vi "practica15RNAtarea.vi"() -> ()   [LabVIEW 2017]
uses:
  <vilib>/Analysis/Matrix/Datatypes/RealMatrix.ctl
  <vilib>/Analysis/Matrix/Numeric/Multiply/Multiply - RM,RM.vi
  <vilib>/Analysis/Matrix/Numeric/Add/Add - RM,RM.vi
  <vilib>/Analysis/Matrix/Numeric/Subtract/Subtract - RM,RM.vi
  <vilib>/Analysis/Matrix/Numeric/Conversions/Matrix To Array - RM.vi
  <vilib>/Analysis/Matrix/NI_Matrix.lvlib
panel:
  out "entrenamiento":bool
  out "Clasificacion":string
  in  "stop":bool
  in  "Ancho":dbl(slide) scale=0.0..200.0
  in  "Alto":dbl(slide) scale=0.0..100.0
  in  "tiempo":dbl(slide) scale=10.0..1000.0
  out "XY Graph":cluster{dbl[], i32[]}[](graph)
  out "Table 2":string[][](table)
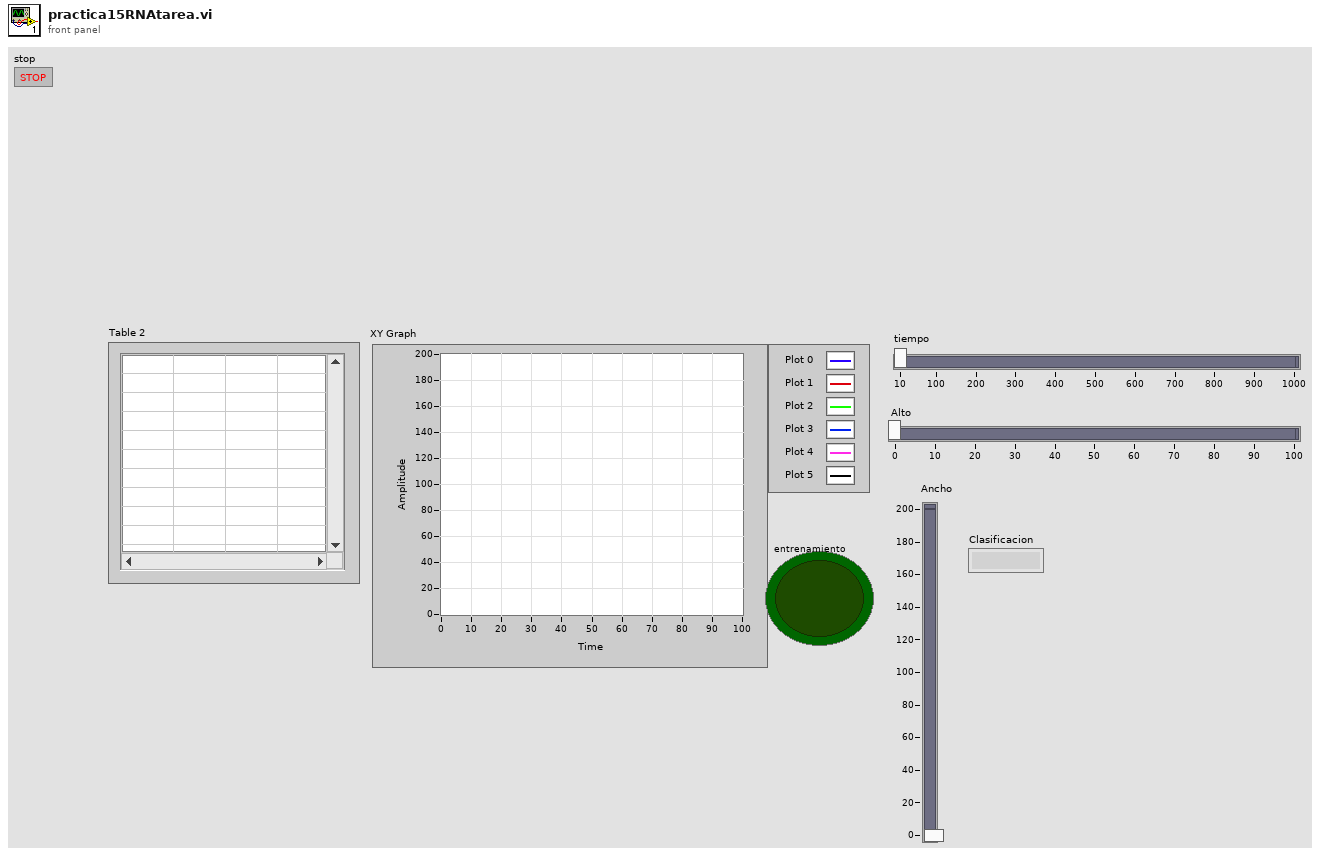
[diagram p1: front panel]
types:
  T1 = typedef "NI_Matrix.lvlib/RealMatrix.ctl" = dbl[][]
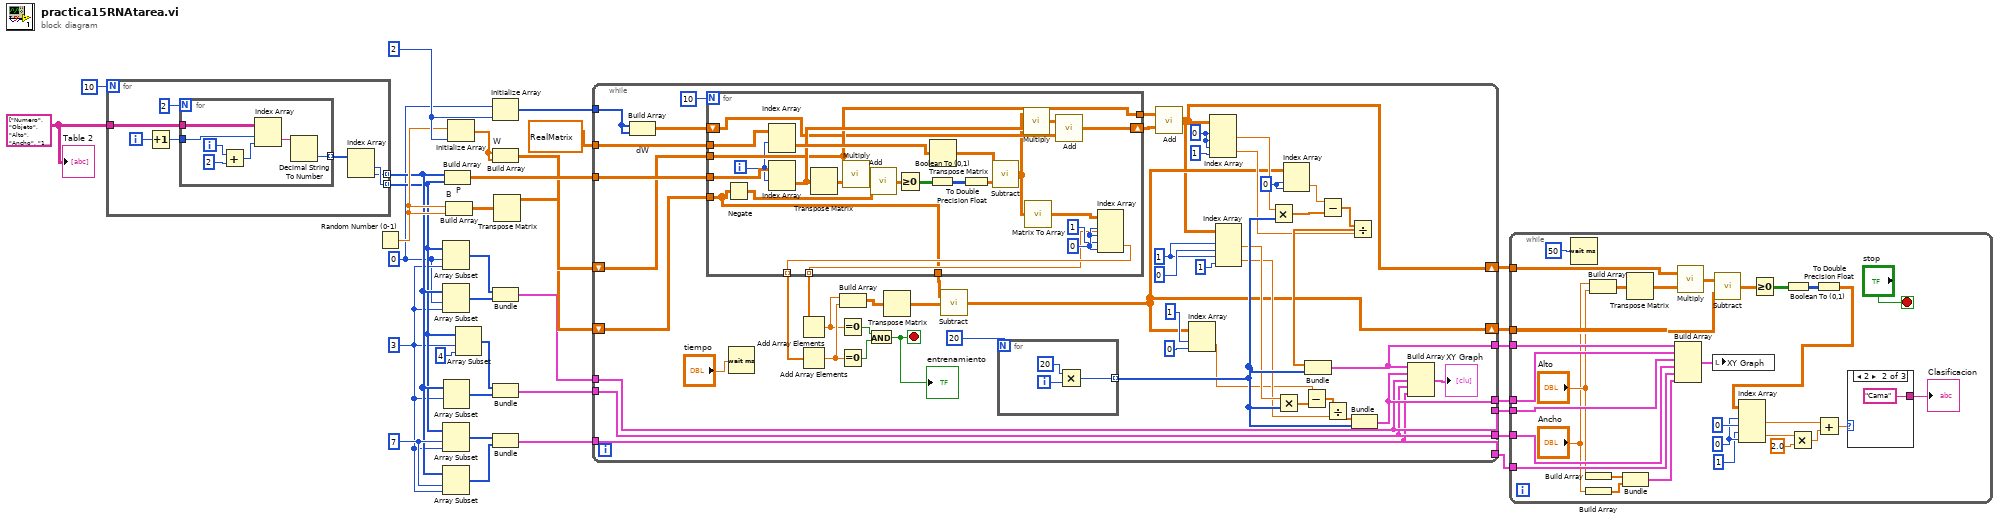
[diagram p0: block diagram]
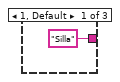
[diagram p2: hidden frame]
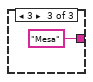
[diagram p3: hidden frame]
diagram:
  w2 = 3 ("length")
  w1 = 0 ("index")
  w22 = 7 ("index")
  w32 = string[][] [["Numero", "Objeto", "Alto", "Ancho"], ["1", "Silla", "40", "48"], ["2", "Silla", "45", "50"], ["3", "Silla", "48", "53"], ["4", "Mesa", "55", "90"], ["5", "Mesa", "60", "80"], ["6", "Mesa", "75", "110"], ["7", "Mesa", "65", "100"], ["8", "Cama", "55", "120"], ["9", "Cama", "48", "140"], ["10", "Cama", "50", "180"]] ("Table")
  w31 = 2 ("dimension size")
  n1 = for {
    N: 10 -> [_]
    tunnel: w32 -> [w38]
    tunnel: [w35] -> w12 mode=indexing
    tunnel: [w34] -> w13 mode=indexing
    i -> [w39]
    n2 = Increment(x=w39) -> (x+1=w37:i32)
    n3 = for {
      N: 2 -> [_]
      tunnel: w37 -> [w42]
      tunnel: w38 -> [w47]
      tunnel: [w43] -> w36 mode=indexing
      i -> [w46]
      n4 = Add(x=w46, y=2) -> (x+y=w41:i32)
      n5 = Index Array(array=w47, index (row)=w42, index (col)=w41) -> (element=w44:string)
      n6 = Decimal String To Number(string=w44) -> (number=w43:i32)  [unwired: 2 in, 1 out]
    }
    n7 = Index Array(array=w36) -> (element #1=w35:i32, element #2=w34:i32)  [unwired: 2 in]
  }
  n8 = Random Number (0-1)() -> (number: 0 to 1=w30:dbl)
  n9 = Array Subset(array=w12, index=w1, length=w2) -> (w16:i32[])
  n10 = Array Subset(array=w13, index=w1, length=w2) -> (w15:i32[])
  n11 = Array Subset(array=w12, index=w22, length=w2) -> (w21:i32[])
  n12 = Array Subset(array=w13, index=w22, length=w2) -> (w20:i32[])
  n13 = Array Subset(array=w13, index=w2) -> (w18:i32[])  [unwired: 1 in]
  n14 = Build Array "P"(w13, w12) -> (w29:T1)
  n15 = Build Array "B"(w30, w30) -> (w27:T1)
  n16 = Initialize Array(w30, w31) -> (w25:dbl[])
  n17 = Array Subset(array=w12, index=w2, length=4) -> (w17:i32[])
  n18 = Initialize Array(w1, w31) -> (w24:i32[])
  n19 = Build Array "W"(w25, w25) -> (w28:T1)
  n20 = Bundle(w16, w15) -> (w10:cluster{i32[], i32[]})  [unwired: 1 in]
  n21 = Bundle(w17, w18) -> (w11:cluster{i32[], i32[]})  [unwired: 1 in]
  n22 = Bundle(w21, w20) -> (w19:cluster{i32[], i32[]})  [unwired: 1 in]
  n23 = Transpose Matrix(1:w27) -> (0:w26:T1)
  n24 = while {
    tunnel: T1 [[1.0, 0.0], [1.0, 0.0], [1.0, 0.0], [1.0, 1.0], [1.0, 1.0], [1.0, 1.0], [1.0, 1.0], [0.0, 1.0], [0.0, 1.0], [0.0, 1.0]] ("T") -> [w93]
    tunnel: w29 -> [w97]
    shift-right: [w50] -> w9
    shift-left: w28 -> [w96]
    shift-right: [w67] -> w8
    shift-left: w26 -> [w94]
    tunnel: w24 -> [w90]
    tunnel: w19 -> [w60]
    tunnel: w11 -> [w61]
    tunnel: w10 -> [w62]
    tunnel: [w64] -> w7
    tunnel: [w63] -> w6
    tunnel: [w62] -> w5
    tunnel: [w61] -> w4
    tunnel: [w60] -> w3
    stop <- w48 stop-if-true
    w75 = 1 ("index (row)")
    w85 = 0 ("index (row)")
    w87 = 0 ("index (row)")
    n25 = Build Array "dW"(w90, w90) -> (w89:T1)
    n26 = for {
      N: 10 -> [_]
      tunnel: w97 -> [w124]
      tunnel: w96 -> [w112]
      tunnel: w94 -> [w101]
      tunnel: w93 -> [w119]
      shift-right: [w115] -> w91
      shift-left: w89 -> [w110]
      tunnel: [w112] -> w92
      tunnel: [w103] -> w54 mode=indexing
      tunnel: [w102] -> w55 mode=indexing
      tunnel: [w101] -> w52
      i -> [w111]
      w114 = 0 ("index (row)")
      n27 = Negate(x=w101) -> (-x=w118:T1)
      n28 = Index Array(array=w119, index (row)=w111) -> (element=w120:T1)  [unwired: 1 in]
      n29 = Index Array(array=w124, index (row)=w111) -> (element=w116:T1)  [unwired: 1 in]
      n30 = Transpose Matrix(1:w116) -> (0:w104:T1)
      n31 = call-poly <vilib>:"Multiply.vi"("Real Matrix B"=w104, "Real Matrix A"=w112) -> ("A * B"=w121:T1)
      n32 = call-poly <vilib>:"Add.vi"("Real Matrix B"=w118, "Real Matrix A"=w121) -> ("A + B"=w109:T1)
      n33 = Greater Or Equal To 0?(x=w109) -> (x >= 0?=w123:bool[][])
      n34 = Boolean To (0,1)(Boolean=w123) -> (0, 1=w122:i16[][])
      n35 = Transpose Matrix(1:w120) -> (0:w108:T1)
      n36 = To Double Precision Float(number=w122) -> (double precision float=w107:dbl[][])
      n37 = call-poly <vilib>:"Subtract.vi"("Real Matrix B"=w107, "Real Matrix A"=w108) -> ("A - B"=w106:T1)
      n38 = call-poly <vilib>:"Multiply.vi"("Real Matrix B"=w116, "Real Matrix A"=w106) -> ("A * B"=w117:T1)
      n39 = call-poly <vilib>:"Matrix To Array.vi"("Real Matrix"=w106) -> ("Real 2D Array"=w105:dbl[][])
      n40 = call-poly <vilib>:"Add.vi"("Real Matrix B"=w110, "Real Matrix A"=w117) -> ("A + B"=w115:T1)
      n41 = Index Array(array=w105, index (row) #1=w114, index (col) #1=w114, index (row) #2=1 ("disabled index (col)"), index (col) #2=w114) -> (element #1=w102:dbl, element #2=w103:dbl)
    }
    n42 = Wait (ms)(milliseconds to wait="tiempo") -> ()  [unwired: 1 out]
    n43 = Add Array Elements(numeric array=w55) -> (sum=w58:dbl)
    n44 = Add Array Elements(numeric array=w54) -> (sum=w59:dbl)
    n45 = Equal To 0?(x=w58) -> (x = 0?=w57:bool)
    n46 = Equal To 0?(x=w59) -> (x = 0?=w56:bool)
    n47 = Build Array(w58, w59) -> (w53:T1)
    n48 = And(x=w57, y=w56) -> (x .and. y?=w48:bool)
    "entrenamiento" <- w48
    n49 = Transpose Matrix(1:w53) -> (0:w51:T1)
    n50 = call-poly <vilib>:"Subtract.vi"("Real Matrix B"=w51, "Real Matrix A"=w52) -> ("A - B"=w67:T1)
    n51 = for {
      N: 20 -> [_]
      tunnel: [w98] -> w78 mode=indexing
      i -> [w99]
      n52 = Multiply(x=20, y=w99) -> (x*y=w98:i32)
    }
    n53 = call-poly <vilib>:"Add.vi"("Real Matrix B"=w91, "Real Matrix A"=w92) -> ("A + B"=w50:T1)
    n54 = Index Array(array=w67, index (row)=1, index (col)=0) -> (element=w70:dbl)
    n55 = Index Array(array=w50, index (row) #1=w87, index (col) #1=w87, index (row) #2=w87, index (col) #2=1 ("index (col)")) -> (element #1=w74:dbl, element #2=w71:dbl)
    n56 = Index Array(array=w50, index (row) #1=w75, index (col) #1=0 ("index (col)"), index (row) #2=w75, index (col) #2=1 ("index (col)")) -> (element #1=w73:dbl, element #2=w72:dbl)
    n57 = Multiply(x=w74, y=w78) -> (x*y=w84:dbl[])
    n58 = Multiply(x=w73, y=w78) -> (x*y=w81:dbl[])
    n59 = Index Array(array=w67, index (row)=w85, index (col)=w85) -> (element=w49:dbl)
    n60 = Subtract(x=w70, y=w81) -> (x-y=w80:dbl[])
    n61 = Subtract(x=w49, y=w84) -> (x-y=w83:dbl[])
    n62 = Divide(x=w80, y=w72) -> (x/y=w79:dbl[])
    n63 = Divide(x=w83, y=w71) -> (x/y=w82:dbl[])
    n64 = Bundle(w82, w78) -> (w64:cluster{dbl[], i32[]})  [unwired: 1 in]
    n65 = Bundle(w79, w78) -> (w63:cluster{dbl[], i32[]})  [unwired: 1 in]
    n66 = Build Array(w64, w63, w62, w61, w60) -> (→"XY Graph":cluster{dbl[], i32[]}[])
  }
  n67 = while {
    tunnel: w9 -> [w141]
    tunnel: w8 -> [w138]
    tunnel: w7 -> [w151]
    tunnel: w6 -> [w150]
    tunnel: w5 -> [w149]
    tunnel: w4 -> [w148]
    tunnel: w3 -> [w147]
    stop <- "stop" stop-if-true
    w133 = 0 ("disabled index (row)")
    n68 = Wait (ms)(milliseconds to wait=u32 50) -> ()  [unwired: 1 out]
    n69 = Build Array("Alto") -> (w154:dbl[])
    n70 = Build Array("Ancho") -> (w155:dbl[])
    n71 = Build Array("Ancho", "Alto") -> (w142:T1)
    n72 = Bundle(w154, w155) -> (w146:cluster{dbl[], dbl[]})  [unwired: 1 in]
    n73 = Transpose Matrix(1:w142) -> (0:w140:T1)
    n74 = Build Array(w151, w150, w149, w148, w147, w146) -> (w145:cluster{dbl[], dbl[]}[])
    n75 = call-poly <vilib>:"Multiply.vi"("Real Matrix B"=w140, "Real Matrix A"=w141) -> ("A * B"=w139:T1)
    n76 = local write "XY Graph"(w145) -> ()
    n77 = call-poly <vilib>:"Subtract.vi"("Real Matrix B"=w138, "Real Matrix A"=w139) -> ("A - B"=w135:T1)
    n78 = Greater Or Equal To 0?(x=w135) -> (x >= 0?=w144:bool[][])
    n79 = Boolean To (0,1)(Boolean=w144) -> (0, 1=w143:i16[][])
    n80 = To Double Precision Float(number=w143) -> (double precision float=w125:dbl[][])
    n81 = Index Array(array=w125, index (row) #1=w133, index (col) #1=0 ("disabled index (col)"), index (row) #2=1 ("disabled index (row)"), index (col) #2=w133) -> (element #1=w129:dbl, element #2=w131:dbl)
    n82 = Multiply(x=w131, y=2.0) -> (x*y=w128:dbl)
    n83 = Add(x=w129, y=w128) -> (x+y=w127:dbl)
    n84 = case shown="2" w127 {
      tunnel: ["Silla" "Cama" "Mesa"] -> w126
      frame 1, Default {
      }
      frame 2 {
      }
      frame 3 {
      }
    }
    "Clasificacion" <- w126
  }
  "Table 2" <- w32
